vi "Move.vi"(0 "Serial Port":refnum<visa-resource-name>="N/A", 1 "Number of Steps":u32, 2 "Direction":bool, 3 "M0":bool, 4 "M1":bool, 5 "error in (no error)":errorcluster) -> (6 "error out":errorcluster)   [LabVIEW 2021]
uses:
  <vilib>/MakerHub/LINX/Public/Peripherals/Digital/Digital Write 1 Chan.vi
  <vilib>/MakerHub/LINX/Public/Peripherals/Digital/Digital Write N Chans.vi
  <vilib>/MakerHub/LINX/Private/Local IO/LinxDigitalWrite.vi
  <vilib>/MakerHub/LINX/Public/Utilities/Check Channel.vi
  <vilib>/MakerHub/LINX/Public/Utilities/Open Serial.vi
  <vilib>/MakerHub/LINX/Private/Utilties/Generate Error.vi
  <vilib>/MakerHub/LINX/LMH-LINX.lvlib
panel:
  out "PIN Step":u8=11
  out "PIN Dir":u8=12
  out "PIN M1":u8=9
  out "PIN M0":u8=8
  out "PIN Sleep":u8=10
  # "Function & M0 & M1\n ----------------------\nFull  Step:       0         0\n1/2   Step:       1         0\n1/8   Step:       0         1\n1/16 Step:       1         1"
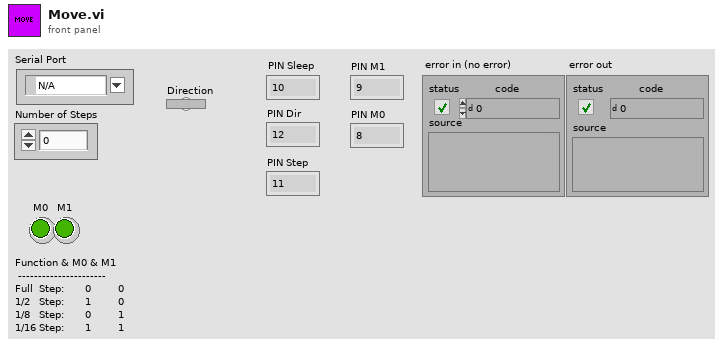
[diagram p1: front panel]
types:
  T1 = typedef "LMH-LINX.lvlib/LINX Ref.ctl" = cluster{"IO":T2, "Interface":T3, "LINX Device Config":T4}
  T2 = typedef "LMH-LINX.lvlib/Platform.ctl" = enum16{"Remote", "Local"}
  T3 = typedef "LMH-LINX.lvlib/Interface.ctl" = enum16{"Serial", "TCP"}
  T4 = typedef "LMH-LINX.lvlib/Device.lvlib/LINX Device Config.ctl" = cluster{"Interface":T3, "COM Port":refnum<visa-resource-name>, "TCP Configuration":T5, "Device Family":u8, "Device ID":u8, "Device Name":string, "TCP Ref":refnum<k5>, "Channels":T6}
  T5 = typedef "LMH-LINX.lvlib/Device.lvlib/TCP Config.ctl" = cluster{"IP Address":string, "Port":u16}
  T6 = typedef "LMH-LINX.lvlib/Channels.ctl" = cluster{"DI":u8[], "DO":u8[], "AI":u8[], "AO":u8[], "PWM":u8[], "QE":u8[], "UART":u8[], "I2C 2":u8[], "SPI":u8[], "CAN":u8[], "Servo":u8[], "AI Ref (V)":dbl, "AI Resolution (Bits)":u8, "AO Ref (V)":dbl, "AO Resolution (Bits)":u8}
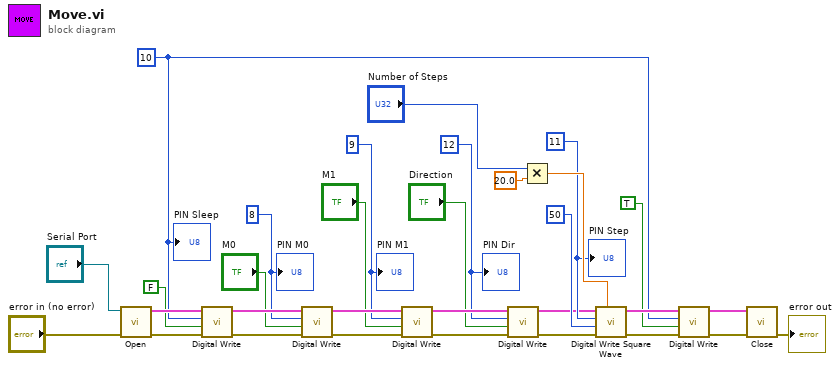
[diagram p0: block diagram]
diagram:
  w18 = u8 12 ("DO Channel")
  w20 = u8 9 ("DO Channel")
  w22 = u8 8 ("DO Channel")
  w12 = u8 10 ("DO Channel")
  w28 = u8 11 ("Channel")
  n1 = call-poly <vilib>:"Open.vi"("Error In"="error in (no error)", "Serial Port"="Serial Port") -> ("Error Out"=w25:errorcluster, "LINX Resource"=w27:T1)  [unwired: 7 in, 1 out]
  n2 = call-poly <vilib>:"Digital Write.vi"("Error In"=w25, "Output Value"=FALSE, "DO Channel"=w12, "LINX Resource"=w27) -> ("Error Out"=w23:errorcluster, "LINX Resource"=w24:T1)  [unwired: 6 in]
  n3 = call-poly <vilib>:"Digital Write.vi"("Error In"=w23, "Output Value"="M0", "DO Channel"=w22, "LINX Resource"=w24) -> ("Error Out"=w17:errorcluster, "LINX Resource"=w21:T1)  [unwired: 6 in]
  n4 = call-poly <vilib>:"Digital Write.vi"("Error In"=w17, "Output Value"="M1", "DO Channel"=w20, "LINX Resource"=w21) -> ("Error Out"=w16:errorcluster, "LINX Resource"=w19:T1)  [unwired: 6 in]
  n5 = call-poly <vilib>:"Digital Write.vi"("Error In"=w16, "Output Value"="Direction", "DO Channel"=w18, "LINX Resource"=w19) -> ("Error Out"=w15:errorcluster, "LINX Resource"=w14:T1)  [unwired: 6 in]
  n6 = Multiply(x="Number of Steps", y=20.0) -> (x*y=w30:dbl)
  n7 = call <vilib>:"Digital Write Square Wave.vi"("Duration (ms)"=w30, "Error In"=w15, "Frequency (Hz)"=u32 50, "Channel"=w28, "LINX Resource"=w14) -> ("Error Out"=w10:errorcluster, "LINX Resource"=w13:T1)  [unwired: 5 in]
  n8 = call-poly <vilib>:"Digital Write.vi"("Error In"=w10, "Output Value"=TRUE, "DO Channel"=w12, "LINX Resource"=w13) -> ("Error Out"=w9:errorcluster, "LINX Resource"=w1:T1)  [unwired: 6 in]
  n9 = call <vilib>:"Close.vi"("Error In"=w9, "LINX Resource"=w1) -> ("Error Out"=→"error out":errorcluster)  [unwired: 9 in]
  "PIN Sleep" <- w12
  "PIN M0" <- w22
  "PIN M1" <- w20
  "PIN Dir" <- w18
  "PIN Step" <- w28
